vi "Check_Traverse_move_PN.vi"(0 "Current position":sgl[](array[numeric])=[0.0, 0.0, 0.0] format="%.2f", 1 "Traverse Name":string, 2 "Full Check":bool, 5 "New Position":sgl[](array[numeric])=[0.0, 0.0, 0.0] format="%.2f", 7 "Model       Roll      Pitch       Yaw (deg)":sgl[](array[numeric]) format="%#.2f", 9 "Traverse Active Parts":cluster{"X":bool, "XY":bool, "XYZ":bool}) -> (6 "Position At Crash":sgl[](array[numeric]) format="%.2f", 10 "Steps":sgl[][](array[numeric]) format="%.2f", 15 "Error Comments":string)   [LabVIEW 2020]
uses:
  Collision_Detection/Triangles/EnFlo specific/Collision Mode.ctl
  Globals/Constants_global.vi
panel:
  # "X                Y                   Z"
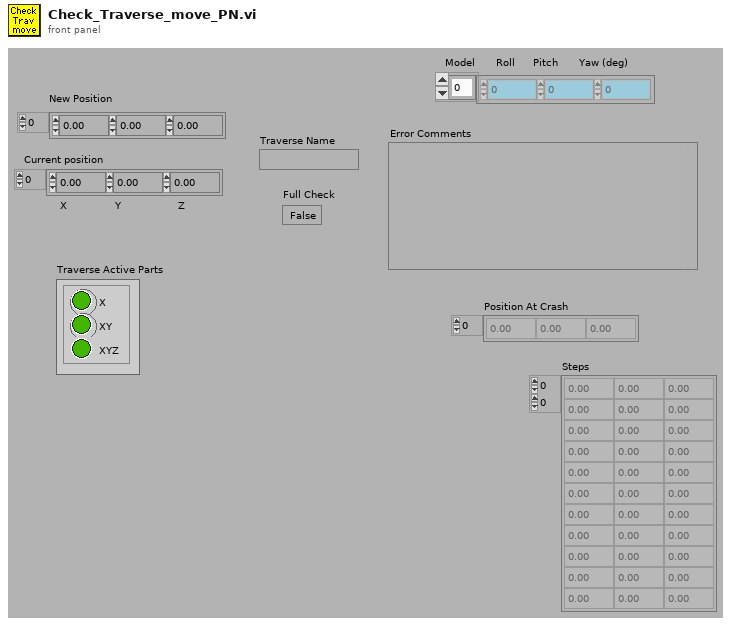
[diagram p1: front panel]
types:
  T1 = enum16{"To Traverse Coordinates", "To User Coordinates"}
  T2 = typedef "Collision Mode.ctl" = enum16{"Traverse - Tunnel", "Traverse - Model", "Traverse - Fixed objects", "Traverse - Traverse", "Traverse - All"}
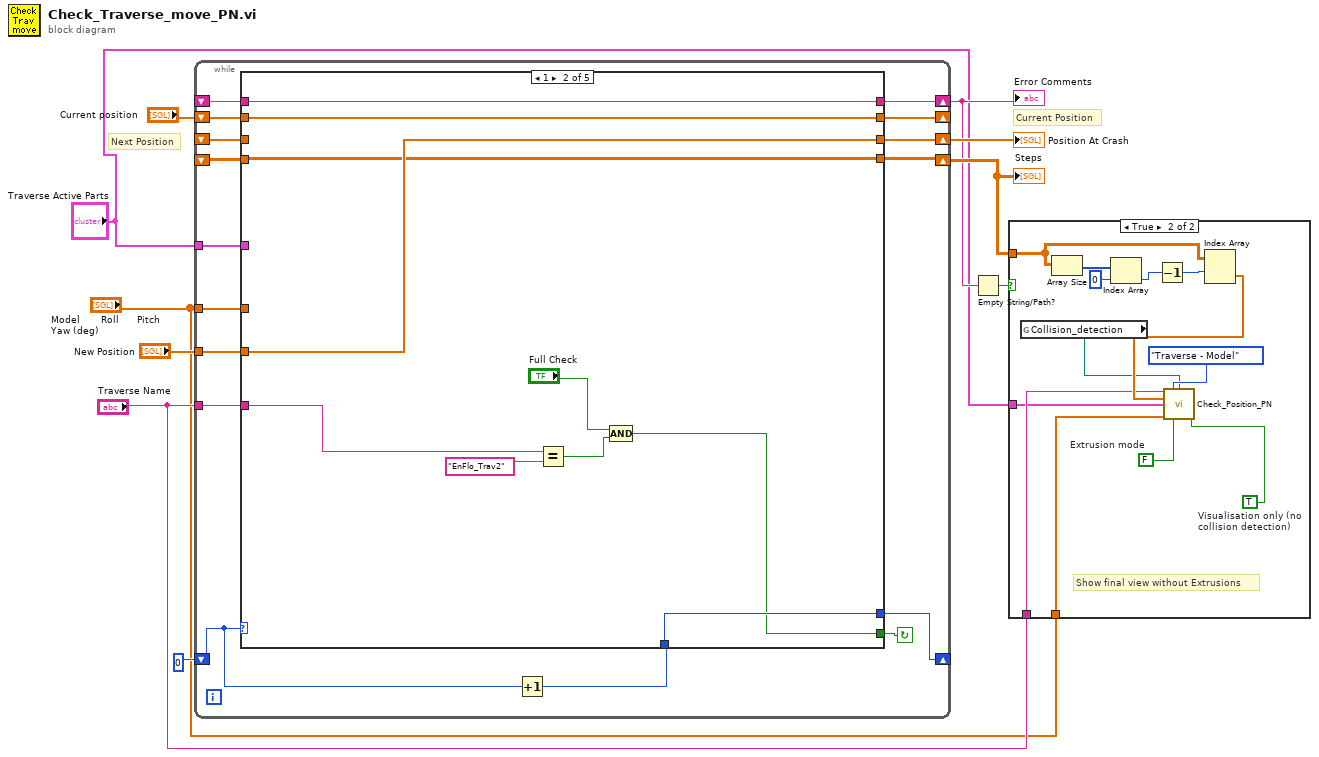
[diagram p0: block diagram]
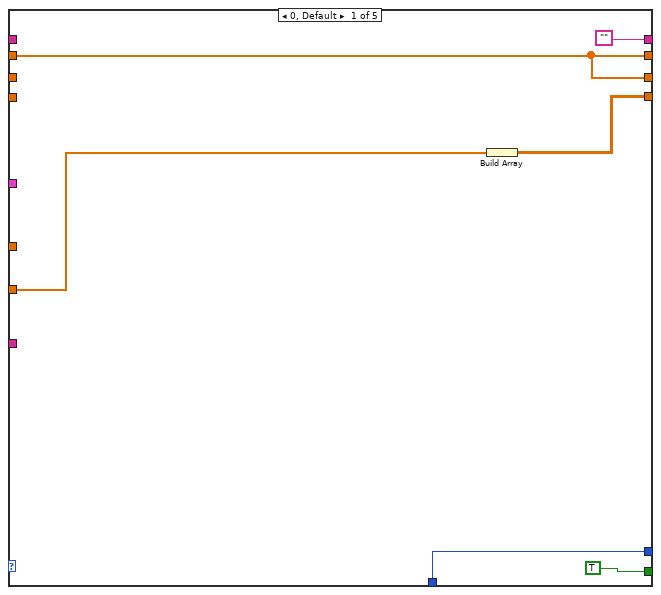
[diagram p3: hidden frame]
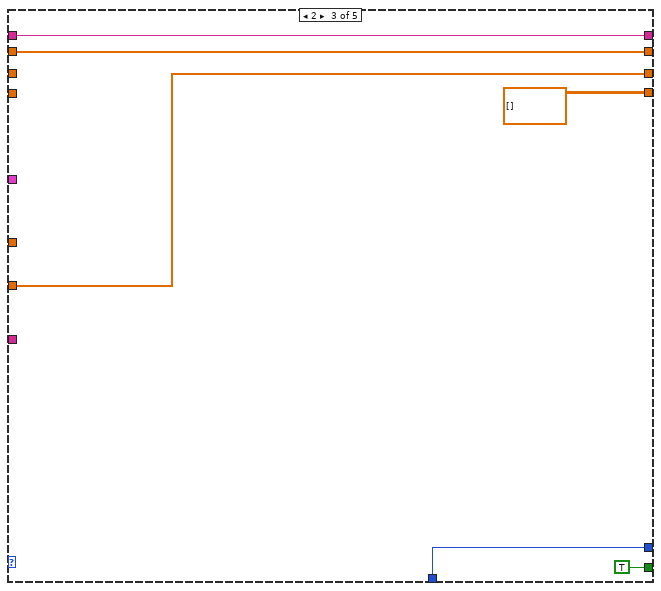
[diagram p4: hidden frame]
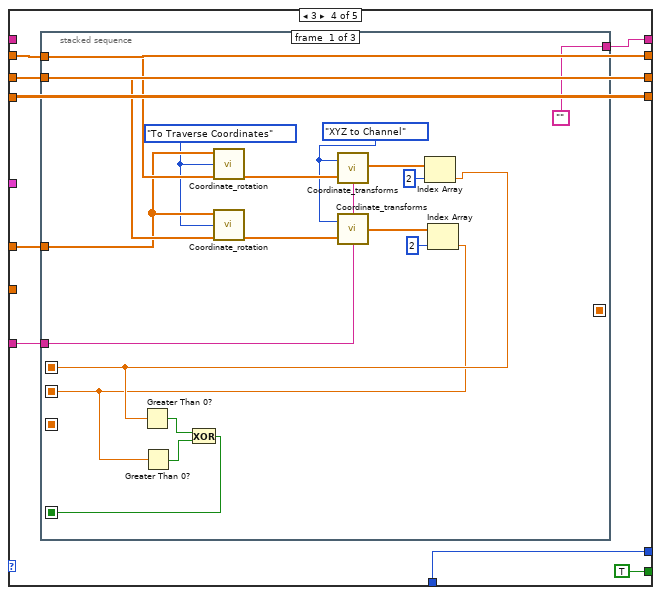
[diagram p5: hidden frame]
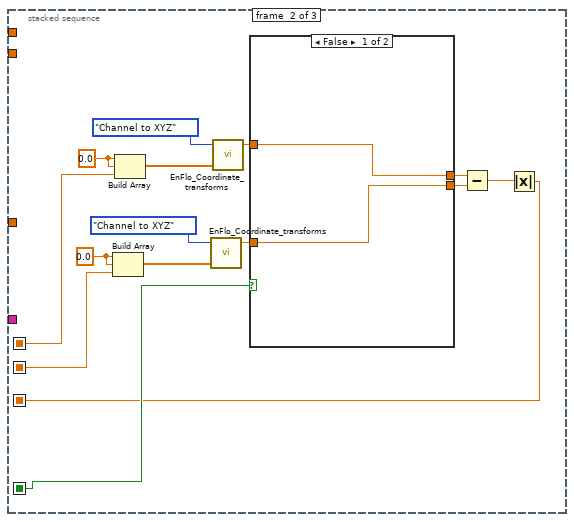
[diagram p6: hidden frame]
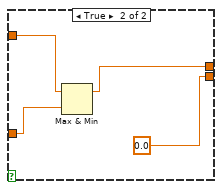
[diagram p7: hidden frame]
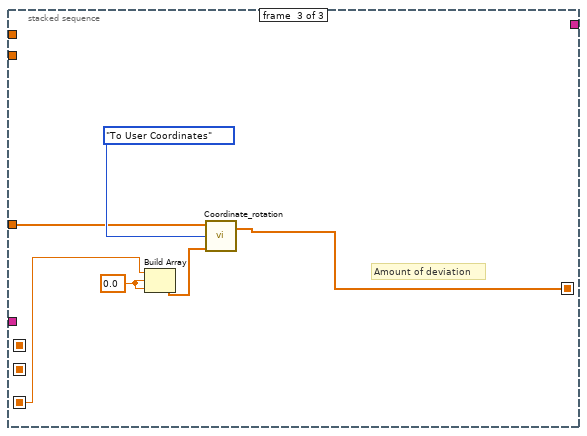
[diagram p8: hidden frame]
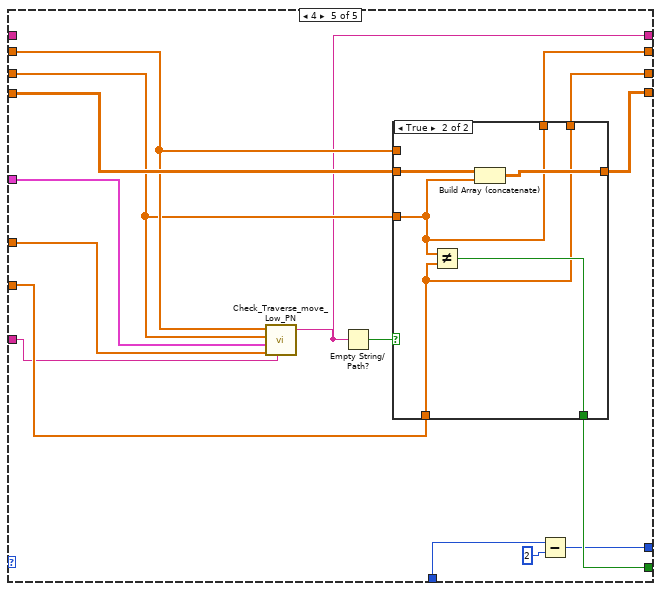
[diagram p9: hidden frame]
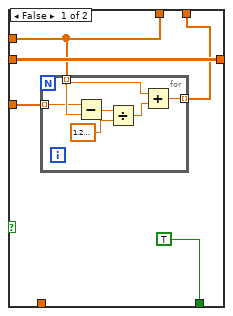
[diagram p10: hidden frame]
diagram:
  # "Current Position"
  # "Next Position"
  n1 = while {
    shift-left: _ -> [w13]
    shift-right: [w12] -> w6
    tunnel: "Model       Roll      Pitch       Yaw (deg)" -> [w14]
    tunnel: "New Position" -> [w15]
    shift-left: _ -> [w17]
    shift-right: [w18] -> w5
    shift-left: 0 -> [w21]
    shift-right: [w20] -> _
    tunnel: "Traverse Name" -> [w22]
    shift-left: _ -> [w16]
    shift-right: [w24] -> w7
    shift-left: "Current position" -> [w26]
    shift-right: [w25] -> _
    tunnel: "Traverse Active Parts" -> [w11]
    stop <- w23 continue-if-true
    n2 = Increment(x=w21) -> (x+1=w19:i32)
    n3 = case shown="1" w21 {
      tunnel: w26 -> [w27 w41 w47 w54 w107]
      tunnel: [w27 w41 w47 w54 w112] -> w25
      tunnel: [w27 w35 w45 w53 w111] -> w24
      tunnel: [TRUE ("Box Inside") w37 TRUE ("Box Inside") TRUE ("Box Inside") w113] -> w23
      tunnel: w22 -> [_ w38 _ w51 w104]
      tunnel: [w29 w40 w46 w50 w109] -> w20
      tunnel: w19 -> [w29 w40 w46 w50 w108]
      tunnel: ["" w42 w48 w56 w103] -> w18
      tunnel: w17 -> [_ w42 w48 _ _]
      tunnel: w16 -> [_ _ _ w53 w106]
      tunnel: w15 -> [w32 w35 w45 _ w114]
      tunnel: w14 -> [_ _ _ w52 w105]
      tunnel: w13 -> [_ w34 _ w49 w117]
      tunnel: [w31 w34 sgl[][] [] w49 w116] -> w12
      tunnel: w11 -> [_ _ _ _ w102]
      frame 0, Default {
        n4 = Build Array(w32) -> (w31:sgl[][])
      }
      frame 1 {
        n5 = Equal?(x=w38, y="EnFlo_Trav2") -> (x = y?=w33:bool)
        n6 = Compound Arithmetic op=AND("Full Check", w33) -> (w37:bool)
      }
      frame 2 {
      }
      frame 3 {
        n7 = stacked-sequence {
          seq-local: [w59 _ _] -> [_ w89 _]
          seq-local: [w58 _ _] -> [_ w88 _]
          seq-local: [w57 _ _] -> [_ w79 _]
          seq-local: [_ w75 _] -> [_ _ w98]
          seq-local: [_ _ w96] -> [_ _ _]
          tunnel: ["" _ _] -> w56
          tunnel: w54 -> [w72 _ _]
          tunnel: w53 -> [w70 _ _]
          tunnel: w52 -> [w69 _ w97]
          tunnel: w51 -> [w68 _ _]
          frame #0 {
            w66 = enum16{"XYZ to Channel", "Channel to XYZ"}."XYZ to Channel" ("Mode")
            w67 = T1."To Traverse Coordinates" ("Mode")
            n8 = call "Coordinate_rotation.vi"("Roll-Pitch-Yaw"=w69, "Input Position"=w72, "Mode"=w67) -> ("Output Position"=w73:sgl[])  [unwired: 2 in, 1 out]
            n9 = call "Coordinate_rotation.vi"("Roll-Pitch-Yaw"=w69, "Input Position"=w70, "Mode"=w67) -> ("Output Position"=w71:sgl[])  [unwired: 2 in, 1 out]
            n10 = call "Coordinate_transforms.vi"("Traverse Name"=w68, "Input"=w73, "Mode"=w66) -> ("Output"=w65:sgl[])
            n11 = call "Coordinate_transforms.vi"("Traverse Name"=w68, "Input"=w71, "Mode"=w66) -> ("Output"=w62:sgl[])
            n12 = Index Array(array=w65, index=2) -> (element=w59:sgl)
            n13 = Greater Than 0?(x=w59) -> (x > 0?=w61:bool)
            n14 = Index Array(array=w62, index=2) -> (element=w58:sgl)
            n15 = Greater Than 0?(x=w58) -> (x > 0?=w60:bool)
            n16 = Exclusive Or(1:w60, 2:w61) -> (0:w57:bool)
          }
          frame #1 {
            w82 = 0.0 ("element")
            w87 = 0.0 ("element")
            n17 = Build Array(w82, w82, w88) -> (w84:dbl[])
            n18 = Build Array(w87, w87, w89) -> (w85:dbl[])
            n19 = call "EnFlo_Coordinate_transforms.vi"("Input"=w84, "Mode"=enum16{"XYZ to Channel", "Channel to XYZ"}."Channel to XYZ") -> ("X theta"=w80:dbl)  [unwired: 3 out]
            n20 = call "EnFlo_Coordinate_transforms.vi"("Input"=w85, "Mode"=enum16{"XYZ to Channel", "Channel to XYZ"}."Channel to XYZ") -> ("X theta"=w81:dbl)  [unwired: 3 out]
            n21 = case shown="False" w79 {
              tunnel: w81 -> [w91 w94]
              tunnel: w80 -> [w90 w95]
              tunnel: [w90 0.0 ("element")] -> w78
              tunnel: [w91 w93] -> w77
              frame False {
              }
              frame True {
                n22 = Max & Min(x=w94, y=w95) -> (max(x,y)=w93:dbl)  [unwired: 1 out]
              }
            }
            n23 = Subtract(x=w77, y=w78) -> (x-y=w76:dbl)
            n24 = Absolute Value(x=w76) -> (abs(x)=w75:dbl)
          }
          frame #2 {
            w100 = 0.0 ("Input Element")
            # "Amount of deviation"
            n25 = Build Array(w98, w100, w100) -> (w99:dbl[])
            n26 = call "Coordinate_rotation.vi"("Roll-Pitch-Yaw"=w97, "Input Position"=w99, "Mode"=T1."To User Coordinates") -> ("Output Position"=w96:sgl[])  [unwired: 2 in, 1 out]
          }
        }
      }
      frame 4 {
        n27 = call "Check_Traverse_move_Low_PN.vi"("Current position"=w107, "New Position"=w106, "Traverse Active Parts"=w102, "Model       Roll      Pitch       Yaw (deg)"=w105, "Traverse Name"=w104) -> ("Error Comments"=w103:string)  [unwired: 2 out]
        n28 = Empty String/Path?(string/path=w103) -> (empty?=w115:bool)
        n29 = case shown="True" w115 {
          tunnel: w117 -> [w122 w133]
          tunnel: [w122 w132] -> w116
          tunnel: w114 -> [_ w130]
          tunnel: [TRUE w131] -> w113
          tunnel: [w120 w129] -> w112
          tunnel: [w118 w130] -> w111
          tunnel: w107 -> [w120 _]
          tunnel: w106 -> [w119 w129]
          frame False {
            n30 = for {
              tunnel: w120 -> [w124] mode=indexing
              tunnel: w119 -> [w123] mode=indexing
              tunnel: [w125] -> w118 mode=indexing
              n31 = Subtract(x=w123, y=w124) -> (x-y=w128:sgl)
              n32 = Divide(x=w128, y=sgl 1.2) -> (x/y=w126:sgl)
              n33 = Add(x=w124, y=w126) -> (x+y=w125:sgl)
            }
          }
          frame True {
            n34 = Not Equal?(x=w129, y=w130) -> (x != y?=w131:bool)
            n35 = Build Array (concatenate)(w133, w129) -> (w132:sgl[][])
          }
        }
        n36 = Subtract(x=w108, y=2) -> (x-y=w109:i32)
      }
    }
  }
  "Error Comments" <- w5
  "Position At Crash" <- w7
  "Steps" <- w6
  n37 = Empty String/Path?(string/path=w5) -> (empty?=w4:bool)
  n38 = case shown="True" w4 {
    tunnel: w6 -> [_ w142]
    tunnel: "Model       Roll      Pitch       Yaw (deg)" -> [_ w139]
    tunnel: "Traverse Name" -> [_ w140]
    tunnel: "Traverse Active Parts" -> [_ w135]
    frame False {
    }
    frame True {
      w137 = FALSE  # Extrusion mode
      w138 = TRUE  # Visualisation only (no collision detection)
      # "Show final view without Extrusions"
      n39 = global read "Constants_global.vi" "Collision_detection"() -> (w134:path)
      n40 = Array Size(array=w142) -> (size(s)=w146:i32[])
      n41 = Index Array(array=w146, index=0) -> (element=w144:i32)
      n42 = Decrement(x=w144) -> (x-1=w143:i32)
      n43 = Index Array(array=w142, index (row)=w143) -> (element=w141:sgl[])  [unwired: 1 in]
      n44 = call "Check_Position_PN.vi"("Traverse Name"=w140, "Collision mode"=Collision_Mode."Traverse - Model", "Collision_detection"=w134, "Position to check"=w141, "Traverse Active Parts"=w135, "Model Rotation (deg)"=w139, "Extrusion mode"=w137, "Visualisation only (no collision detection)"=w138) -> ()  [unwired: 3 in, 5 out]
    }
  }
